vi "Create Message Channels.vi"(6 "VS channel direction":T1, 8 "error in (no error)":errorcluster, 10 "Parameters":T2(array[cluster]), 11 "Data Words section in":T3=18446744073709551615 format="%.0x") -> (0 "error out":errorcluster, 3 "Data Words section out":T3=18446744073709551615 format="%.0x")   [LabVIEW 2020, in "Ballard 1553 System Explorer.lvlib"]
uses:
  Ballard 1553 System Explorer.lvlib
  <vilib>/NI VeriStand/Custom Device API/Custom Device Item Ref.ctl
  <vilib>/NI VeriStand/Custom Device API/Custom Device Channel Type.ctl
  <vilib>/NI VeriStand/Custom Device API/Custom Device Channel.ctl
  <vilib>/NI VeriStand/Custom Device API/Custom Device API.lvlib
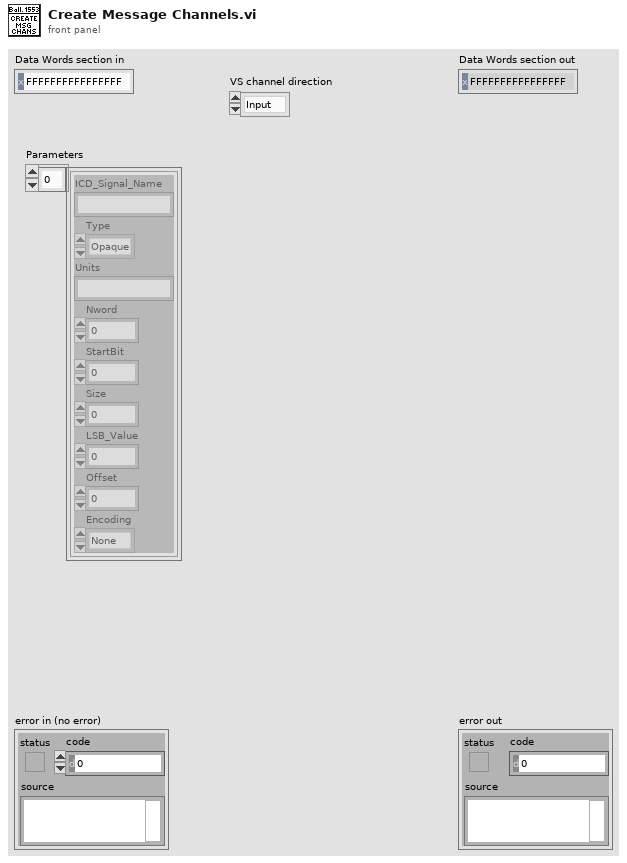
[diagram p1: front panel]
types:
  T1 = typedef "Custom Device API.lvlib/Custom Device Channel Type.ctl" = enum16{"Input", "Output"}
  T2 = cluster{"ICD_Signal_Name":string, "Type":enum16{"Opaque", "Enum", "Float", "Integer", "Bcd", "Bool"}, "Units":string, "Nword":i32, "StartBit":i32, "Size":i32, "LSB_Value":i32, "Offset":i32, "Encoding":enum16{"None", "2-complement", "Unsigned"}}[]
  T3 = typedef "Custom Device API.lvlib/Custom Device Item Ref.ctl" = u64
  T4 = typedef "Custom Device API.lvlib/Custom Device Channel.ctl" = cluster{"Type":T1, "Units":string, "Default Value":dbl, "Faultable":bool, "Scalable":bool}
  T5 = enum16{"Opaque", "Enum", "Float", "Integer", "Bcd", "Bool"}
  T6 = typedef "Custom Device API.lvlib/Custom Device Item Info.ctl" = cluster{"Name":string, "Is Channel":bool, "GUID":string, "Is Waveform":bool}
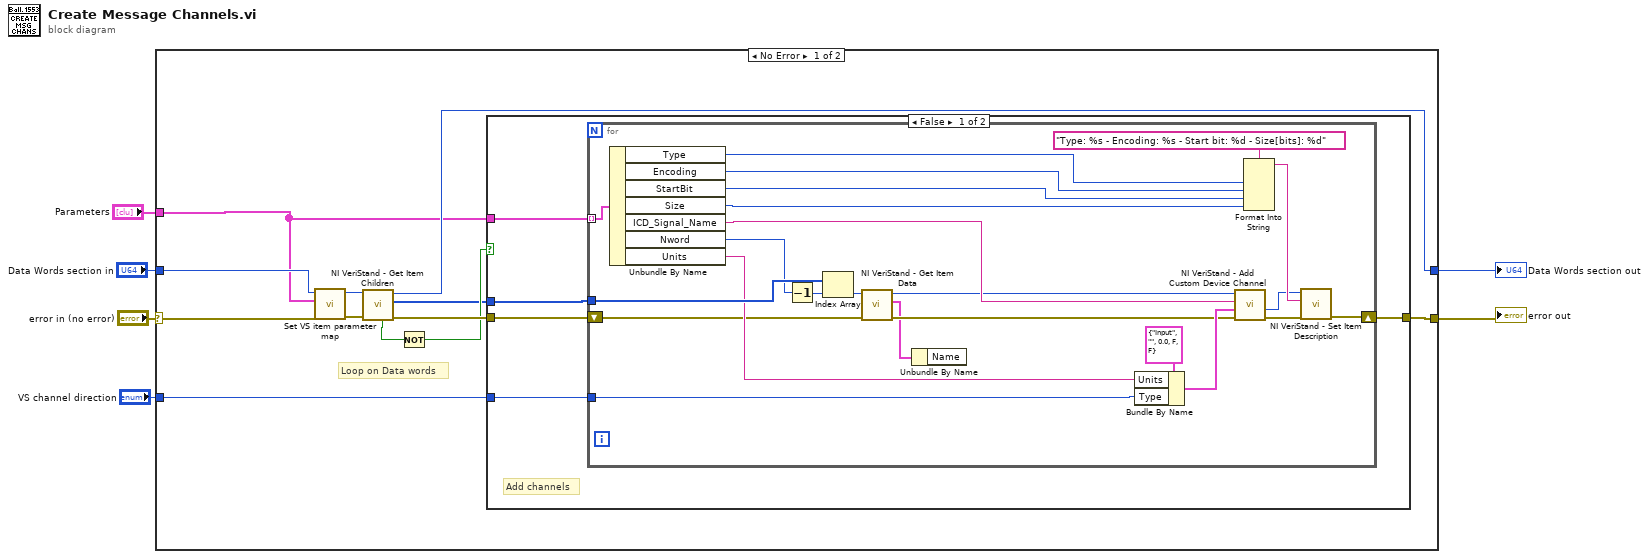
[diagram p0: block diagram]
diagram:
  n1 = case shown="No Error" "error in (no error)" {
    selector: "error in (no error)" -> [w12 w48]
    tunnel: "Data Words section in" -> [w13 w49]
    tunnel: [w14 w49] -> w4
    tunnel: [w18 w48] -> w3
    tunnel: "VS channel direction" -> [w9 _]
    tunnel: "Parameters" -> [w7 _]
    frame No Error {
      # "Loop on Data words"
      n2 = call "Set VS item parameter map.vi"("error in (no error)"=w12, "param config in"=w7, "Iten refs in"=w13) -> ("error out"=w11:errorcluster, "Iten refs out"=w10:T3)  [unwired: 6 in, 1 out]
      n3 = call <vilib>:"NI VeriStand - Get Item Children.vi"("error in (no error)"=w11, "Item Ref in"=w10) -> ("error out"=w17:errorcluster, "Child Refs"=w8:T3[], "Item Ref out"=w14:T3, "Found"=w16:bool)  [unwired: 6 in]
      n4 = Not(x=w16) -> (.not. x?=w15:bool)
      n5 = case shown="False" w15 {
        tunnel: [w20 w47] -> w18
        tunnel: w17 -> [w23 w47]
        tunnel: w8 -> [w22 _]
        tunnel: w7 -> [w21 _]
        tunnel: w9 -> [w19 _]
        frame False {
          # "Add channels"
          n6 = for {
            tunnel: w22 -> [w45]
            tunnel: w21 -> [w46] mode=indexing
            shift-right: [w37] -> w20
            shift-left: w23 -> [w31]
            tunnel: w19 -> [w40]
            n7 = Unbundle By Name(w46) -> ("Type"=w36:T5, "Encoding"=w35:enum16{"None", "2-complement", "Unsigned"}, "StartBit"=w25:i32, "Size"=w24:i32, "ICD_Signal_Name"=w32:string, "Nword"=w44:i32, "Units"=w39:string)
            n8 = Decrement(x=w44) -> (x-1=w43:i32)
            n9 = Index Array(array=w45, index=w43) -> (element=w30:T3)
            n10 = call <vilib>:"NI VeriStand - Get Item Data.vi"("error in (no error)"=w31, "Item Ref in"=w30) -> ("error out"=w29:errorcluster, "Item Info"=w27:T6, "Item Ref out"=w28:T3)  [unwired: 7 out]
            n11 = Unbundle By Name(w27) -> ()  [unwired: 1 out]
            n12 = Bundle By Name(cluster=T4 {"Type"=enum."Input", "Units"="", "Default Value"=0.0, "Faultable"=FALSE, "Scalable"=FALSE} ("Channel"), "Units"=w39, "Type"=w40) -> (w41:T4)
            n13 = call <vilib>:"NI VeriStand - Add Custom Device Channel.vi"("error in (no error)"=w29, "Channel"=w41, "Channel Name"=w32, "Parent Ref in"=w28) -> ("error out"=w38:errorcluster, "Channel Ref"=w26:T3)  [unwired: 4 in, 2 out]
            n14 = Format Into String(format string="Type: %s - Encoding: %s - Start bit: %d - Size[bits]: %d", w36, w35, w25, w24) -> (resulting string=w33:string)  [unwired: 2 in, 1 out]
            n15 = call <vilib>:"NI VeriStand - Set Item Description.vi"("error in (no error)"=w38, "Description"=w33, "Item Ref in"=w26) -> ("error out"=w37:errorcluster)  [unwired: 6 in, 2 out]
          }
        }
        frame True {
          # "No key or no DW, do nothing"
        }
      }
    }
    frame Error {
    }
  }
  "error out" <- w3
  "Data Words section out" <- w4
